vi "Data Storage.vi"(8 "error in (no error)":errorcluster, 10 "Data In":u16[](array[numeric]), 11 "Circular Buffer 1D U16 DVR Queue in":refnum<class "Circular Buffer 1D U16 DVR Queue.lvclass">) -> (0 "error out":errorcluster, 3 "Circular Buffer 1D U16 DVR Queue out":refnum<class "Circular Buffer 1D U16 DVR Queue.lvclass">)   [LabVIEW 2019, in "Circular Buffer 1D U16 DVR Queue.lvclass"]
uses:
  Circular Buffer 1D U16 DVR Queue.lvclass
  Circular Buffer 1D U16 DVR Queue.lvclass/Circular Buffer 1D U16 DVR Queue.ctl
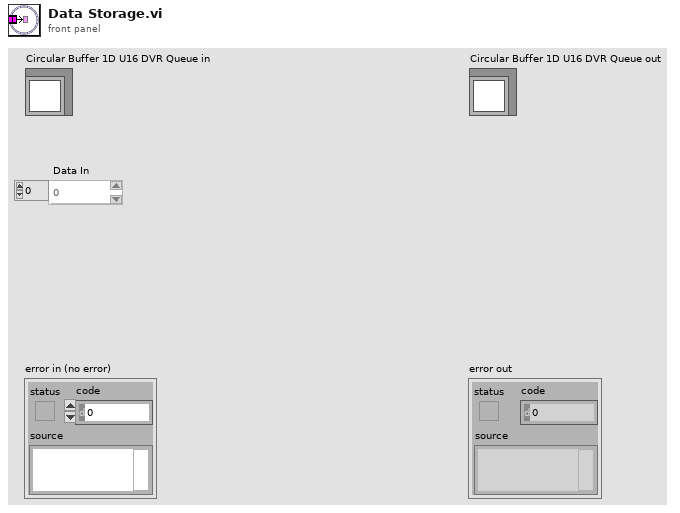
[diagram p1: front panel]
types:
  T1 = typedef "1D U16 DVR Queue.ctl" = refnum<queue>
  T2 = typedef "1D U16 DVR.ctl" = refnum<data-value>
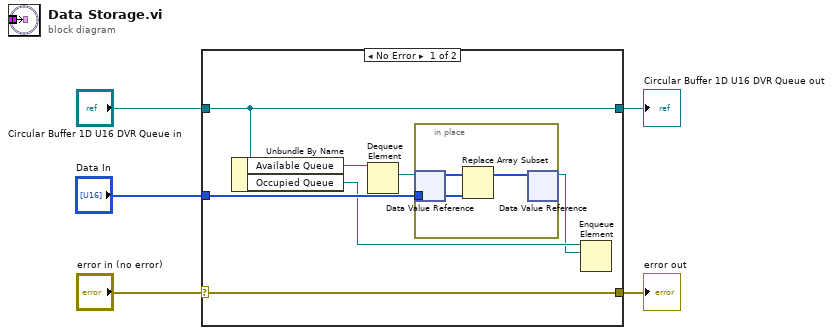
[diagram p0: block diagram]
diagram:
  n1 = case shown="No Error" "error in (no error)" {
    selector: "error in (no error)" -> [w12 w17]
    tunnel: [w12 w17] -> w4
    tunnel: [w11 w16] -> w2
    tunnel: "Circular Buffer 1D U16 DVR Queue in" -> [w11 w16]
    tunnel: "Data In" -> [w8 _]
    frame No Error {
      n2 = Unbundle By Name(w11) -> ("Available Queue"=w10:T1, "Occupied Queue"=w7:T1)
      n3 = Dequeue Element(queue=w10) -> (element=w9:T2)  [unwired: 2 in, 3 out]
      n4 = in-place {
        in-place-border: w8 -> [w13]
        n5 = in-place-dvr #1(w9) -> (w15:u16[])  [unwired: 1 out]
        n6 = Replace Array Subset(array=w15, new element=w13) -> (w14:u16[])  [unwired: 1 in]
        n7 = in-place-dvr #1(w14) -> (w6:T2)  [unwired: 1 out]
      }
      n8 = Enqueue Element(queue=w7, element=w6) -> ()  [unwired: 2 in, 3 out]
    }
    frame Error {
    }
  }
  "error out" <- w4
  "Circular Buffer 1D U16 DVR Queue out" <- w2
